vi "未命名 2.vi"() -> ()   [LabVIEW 2013]
uses:
  <vilib>/Utility/miscctls.llb/LVPoint32TypeDef.ctl
  <vilib>/Utility/miscctls.llb/LVRowAndColumnTypeDef.ctl
panel:
  out "单元格位置":T1
  out "项标识符":string
  out "坐标":T2
  in  "多列列表框":i32(listbox)
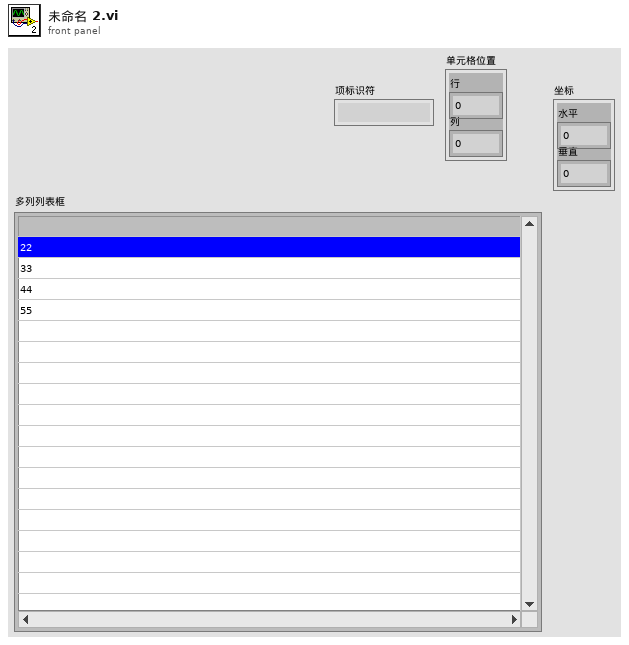
[diagram p1: front panel]
types:
  T1 = typedef "LVRowAndColumnTypeDef.ctl" = cluster{"Row":i32, "Column":i32}
  T2 = typedef "LVPoint32TypeDef.ctl" = cluster{"Horizontal":i32, "Vertical":i32}
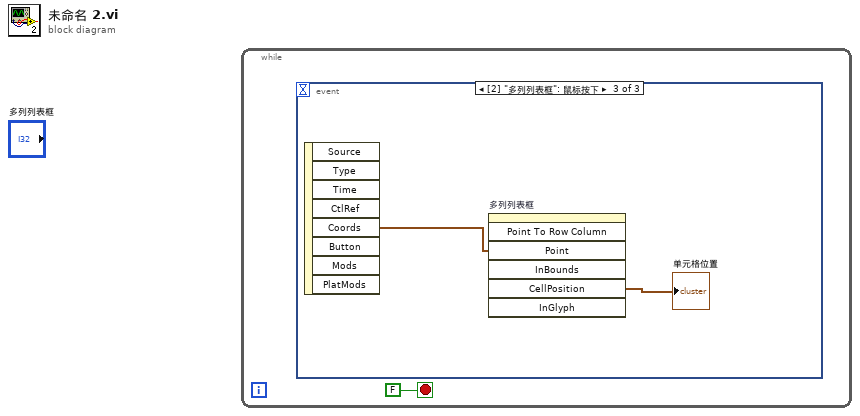
[diagram p0: block diagram]
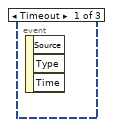
[diagram p2: hidden frame]
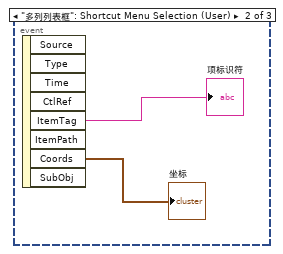
[diagram p3: hidden frame]
diagram:
  n1 = while {
    stop <- FALSE stop-if-true
    n2 = event shown="[2] \"多列列表框\": 鼠标按下" {
      selector: _ -> [_ _ _]
      dyn-events: _ -> [_ _ _]
      timeout: _ -> [_ _ _]
      event Timeout {
        n3 = event-data() -> ()  [unwired: 1 in, 3 out]
      }
      event "多列列表框": Shortcut Menu Selection (User) {
        n4 = event-data() -> ("ItemTag"=→"项标识符":string, "Coords"=→"坐标":T2)  [unwired: 1 in, 6 out]
      }
      event "多列列表框": Mouse Down {
        n5 = event-data() -> ("Coords"=w5:T2)  [unwired: 1 in, 7 out]
        n6 = invoke on="多列列表框" class="MCListbox (严格)" method="Point To Row Column"("Point"=w5) -> ("CellPosition"=→"单元格位置":T1)  [unwired: 6 in, 6 out]
      }
    }
  }
